vi "Motor_Lumicks_MengRonen.vi"() -> ()   [LabVIEW 2014]
uses:
  <vilib>/userdefined/High Color/IMAQdx.ctl
  <vilib>/Utility/inputDevices.llb/joystickAcquire.vi
  <vilib>/Utility/inputDevices.llb/closeJoystick.vi
  <vilib>/vision/driver/NI_Vision_Acquisition_Software.lvlib
panel:
  out "0 Position":T1={"X Pos (mm)"=2.683244, "Y Pos (mm)"=-0.037109375, "Z Pos (mm)"=0.2016383} {"Y Pos (mm)" format="%.3f"; "Z Pos (mm)" format="%.3f"; "X Pos (mm)" format="%.3f"}
  out "error out 2":errorcluster
  out "Image":T2(plugin-control)
  in  "Goto Channel 5":bool
  in  "Goto Channel 4":bool
  in  "Capture Channel 5":bool
  in  "Capture Channel 4":bool
  out "Channel 5":T1={"X Pos (mm)"=0.00014575559, "Y Pos (mm)"=-0.0013701026, "Z Pos (mm)"=0.004635028} {"Y Pos (mm)" format="%.3f"; "Z Pos (mm)" format="%.3f"; "X Pos (mm)" format="%.3f"}
  out "Channel 4":T1={"X Pos (mm)"=0.00014575559, "Y Pos (mm)"=-0.0013701026, "Z Pos (mm)"=0.004635028} {"Y Pos (mm)" format="%.3f"; "Z Pos (mm)" format="%.3f"; "X Pos (mm)" format="%.3f"}
  in  "Stop All":bool=TRUE
  out "button 4":bool
  in  "button 3":bool
  in  "Motor Cruise Param":T3={"X Acc (mm/s^2)"=0.1, "X Vmax (mm/s)"=1.0, "Y Acc (mm/s^2)"=0.3, "Y Vmax (mm/s)"=1.0, "Z Acc (mm/s^2)"=0.1, "Z Vmax (mm/s)"=0.1}
  out "XYZ position":sgl[](array[numeric])=[1.7793261, 1.7925023, 3.857043]
  in  "Motor Limits":T4={"XMAX"=12.0, "XMIN"=-12.0, "YMAX"=12.0, "YMIN"=-12.0, "ZMAX"=10.0, "ZMIN"=-10.0}
  in  "Motor settings (X,Y)":cluster{"Vmax (mm/s)":sgl, "Acc (mm/s/s)":sgl}={"Vmax (mm/s)"=0.05, "Acc (mm/s/s)"=0.2}
  in  "Motor settings (Z)":cluster{"Vmax (mm/s)":sgl, "Acc (mm/s/s)":sgl}={"Vmax (mm/s)"=0.02, "Acc (mm/s/s)"=0.2}
  in  "Capture Channel 3":bool
  in  "Capture Channel 2":bool
  in  "Capture Channel 1":bool
  in  "Goto Channel 2":bool
  in  "Goto Channel 3":bool
  in  "Goto Channel 1":bool
  out "Channel 1":T1={"X Pos (mm)"=2.683244, "Y Pos (mm)"=-0.037109375, "Z Pos (mm)"=0.2016383} {"Y Pos (mm)" format="%.3f"; "Z Pos (mm)" format="%.3f"; "X Pos (mm)" format="%.3f"}
  out "Channel 2":T1={"X Pos (mm)"=2.3714144, "Y Pos (mm)"=-0.4775245, "Z Pos (mm)"=0.20615672} {"Y Pos (mm)" format="%.3f"; "Z Pos (mm)" format="%.3f"; "X Pos (mm)" format="%.3f"}
  out "Channel 3":T1={"X Pos (mm)"=3.6928055, "Y Pos (mm)"=-0.788188, "Z Pos (mm)"=0.19962686} {"Y Pos (mm)" format="%.3f"; "Z Pos (mm)" format="%.3f"; "X Pos (mm)" format="%.3f"}
  out "error out":errorcluster
  in  "MG17Motor Z":refnum<k7>(container)
  in  "MG17Motor Y":refnum<k7>(container)
  in  "MG17Motor X":refnum<k7>(container)
  out "Stage Moving":bool
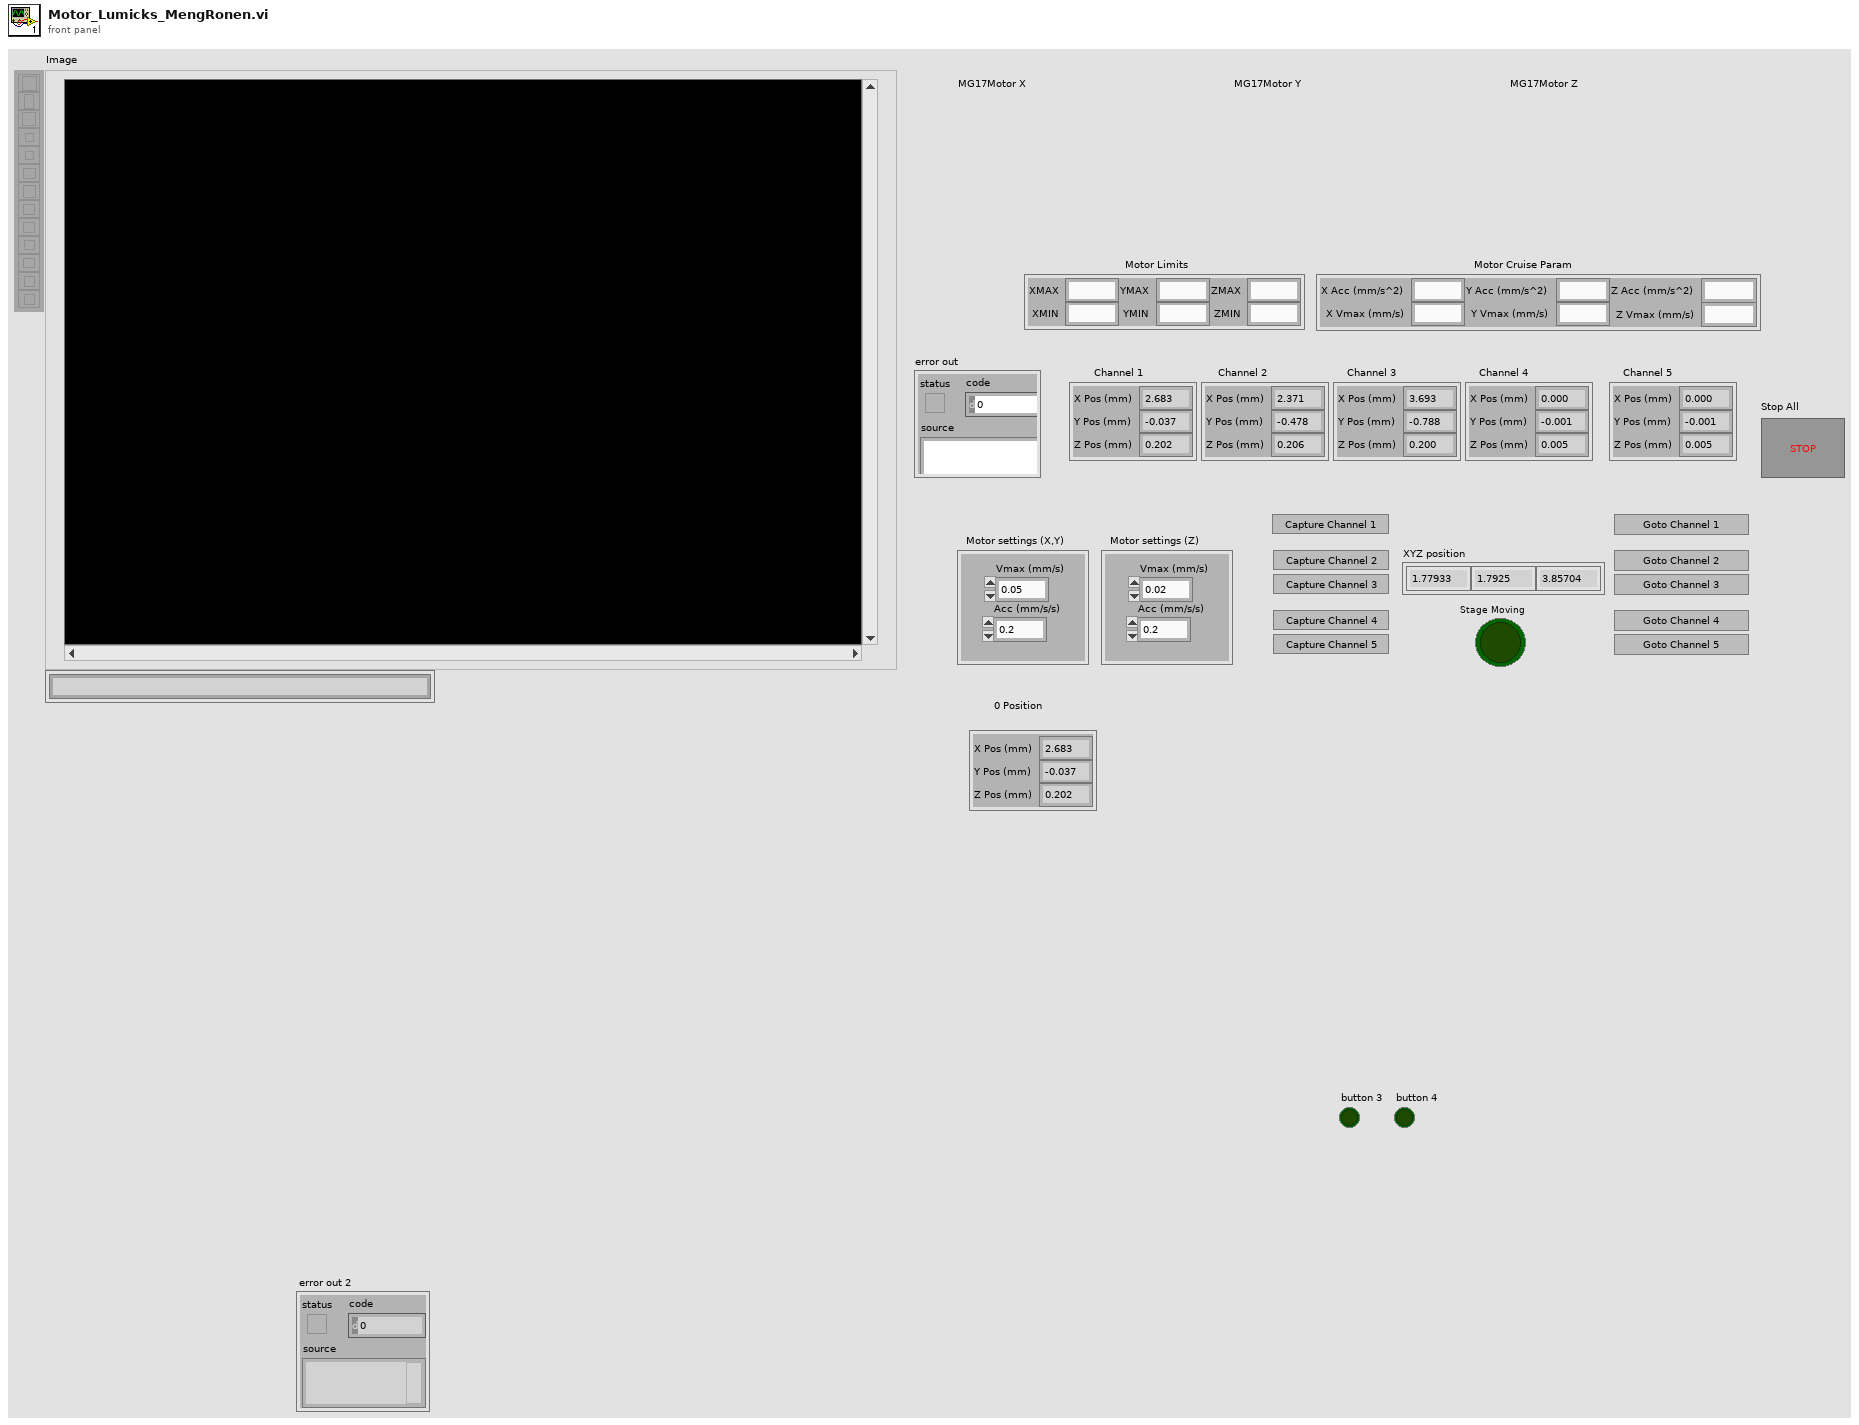
[diagram p1: front panel]
types:
  T1 = cluster{"X Pos (mm)":sgl, "Y Pos (mm)":sgl, "Z Pos (mm)":sgl}
  T2 = typedef "IMAQ Image.ctl" = refnum<image>
  T3 = cluster{"X Acc (mm/s^2)":sgl, "X Vmax (mm/s)":sgl, "Y Acc (mm/s^2)":sgl, "Y Vmax (mm/s)":sgl, "Z Acc (mm/s^2)":sgl, "Z Vmax (mm/s)":sgl}
  T4 = cluster{"XMAX":sgl, "XMIN":sgl, "YMAX":sgl, "YMIN":sgl, "ZMAX":sgl, "ZMIN":sgl}
  T5 = typedef "IMAQdx.ctl" = refnum<k21>
  T6 = typedef "Image Type" = u32
  T7 = cluster{"X axis":i32, "Y axis":i32, "Z axis":i32, "X axis rotation":i32, "Y axis rotation":i32, "Z axis rotation":i32, "U axis":i32, "V axis":i32}
  T8 = cluster{"button 1":bool, "button 2":bool, "button 3":bool, "button 4":bool, "button 5":bool, "button 6":bool, "button 7":bool, "button 8":bool, "button 9":bool, "button 10":bool, "button 11":bool, "button 12":bool, "button 13":bool, "button 14":bool, "button 15":bool, "button 16":bool, "button 17":bool, "button 18":bool, "button 19":bool, "button 20":bool, "button 21":bool, "button 22":bool, "button 23":bool, "button 24":bool, "button 25":bool, "button 26":bool, "button 27":bool, "button 28":bool, "button 29":bool, "button 30":bool, "button 31":bool, "button 32":bool}
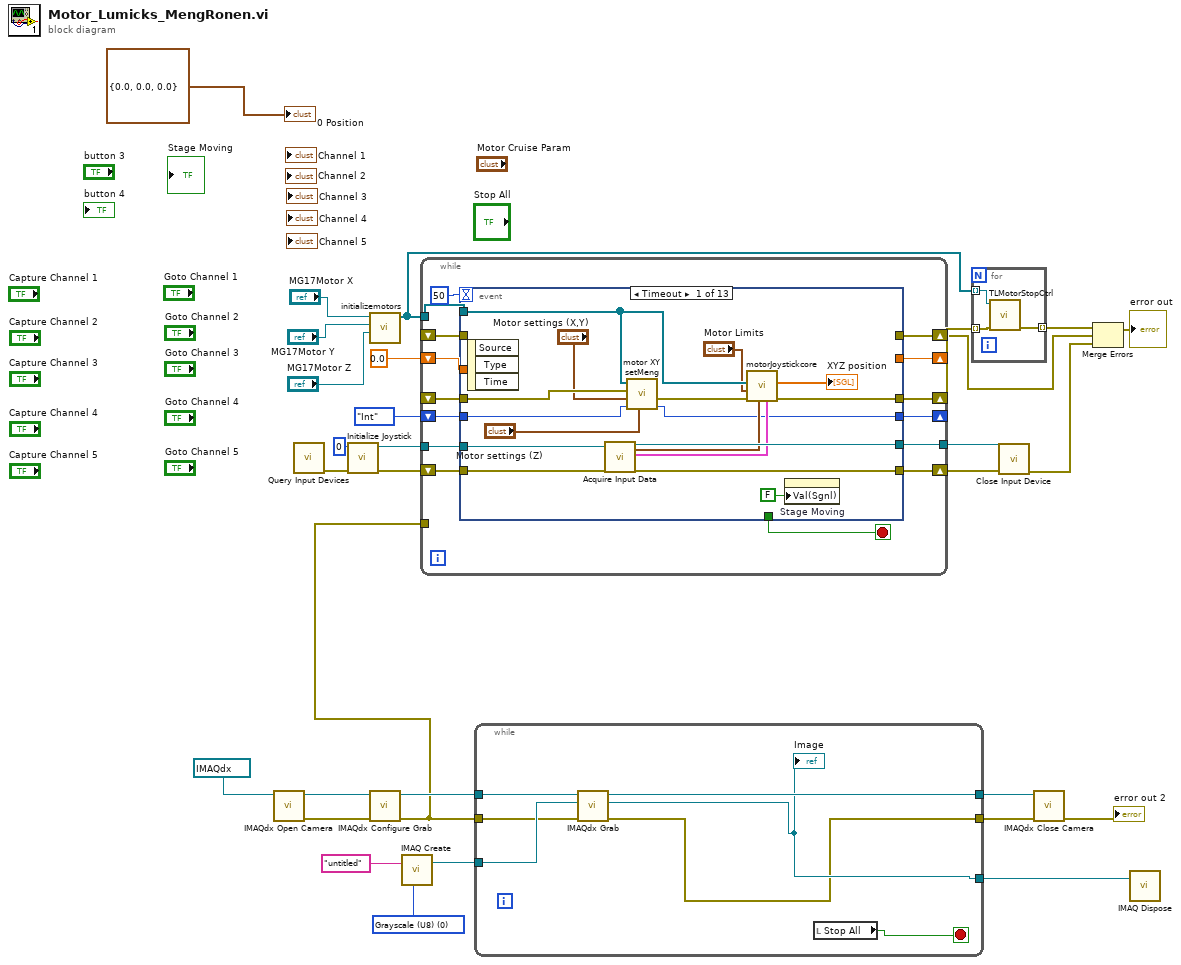
[diagram p0: block diagram]
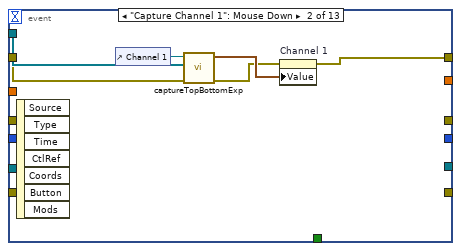
[diagram p2: hidden frame]
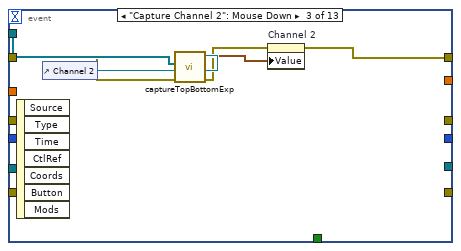
[diagram p3: hidden frame]
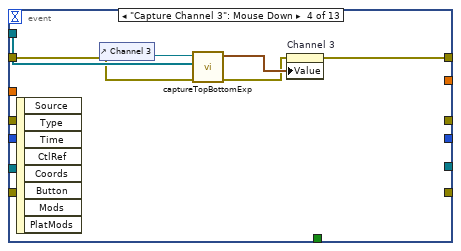
[diagram p4: hidden frame]
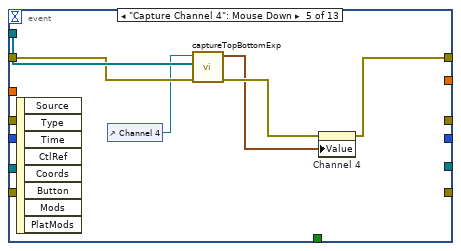
[diagram p5: hidden frame]
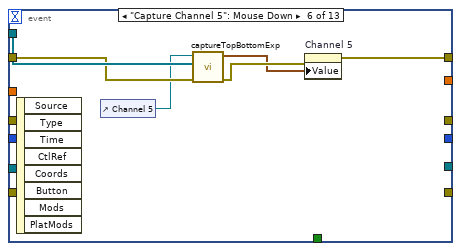
[diagram p6: hidden frame]
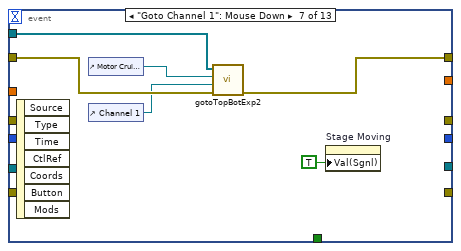
[diagram p7: hidden frame]
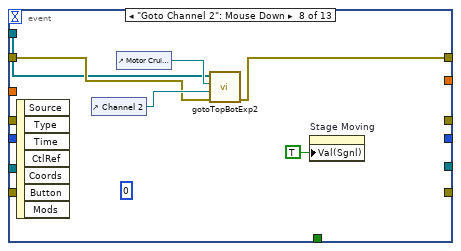
[diagram p8: hidden frame]
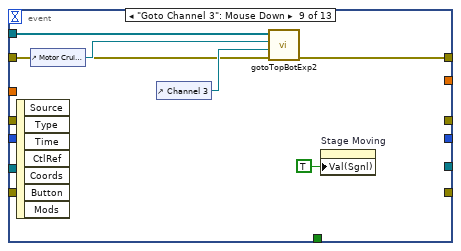
[diagram p9: hidden frame]
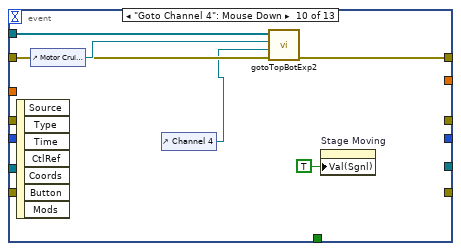
[diagram p10: hidden frame]
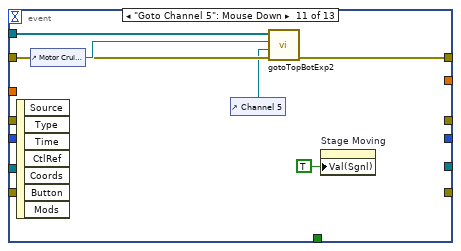
[diagram p11: hidden frame]
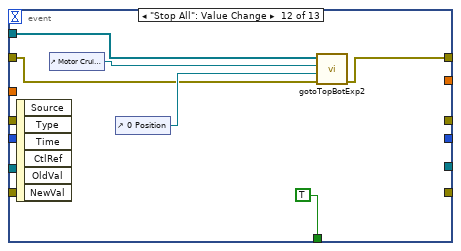
[diagram p12: hidden frame]
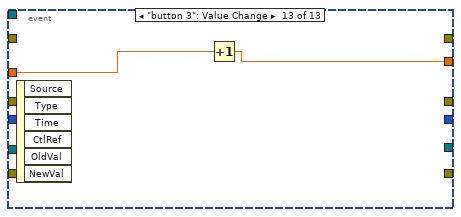
[diagram p13: hidden frame]
diagram:
  w7 = T6 0 items=["Grayscale (U8)", "Grayscale (I16)", "Grayscale (SGL)", "Complex (CSG)", "RGB (U32)", "HSL (U32)", "RGB (U64)", "Grayscale (U16)"] ("Image Type")
  n1 = call <vilib>:"IMAQdx Open Camera.vi"("Session In"=T5 "cam0") -> ("error out"=w11:errorcluster, "Session Out"=w10:T5)  [unwired: 9 in]
  n2 = call <vilib>:"Query Input Devices.vi"() -> ("error out"=w23:errorcluster)  [unwired: 8 in, 3 out]
  n3 = call <vilib>:"Initialize Joystick.vi"("error in (no error)"=w23, "device index"=0) -> ("error out"=w20:errorcluster, "device ID"=w21:refnum<k1>)  [unwired: 8 in]
  n4 = call "initializemotors.vi"("MG17Motor Z"="MG17Motor Z", "MG17Motor Y"="MG17Motor Y", "Automation Refnum in"="MG17Motor X") -> ("Array 2"=w25:refnum<k7>[])  [unwired: 7 in, 1 out]
  n5 = call <vilib>:"IMAQdx Configure Grab.vi"("error in"=w11, "Session In"=w10) -> ("error out"=w2:errorcluster, "Session Out"=w9:T5)  [unwired: 8 in]
  n6 = call "IMAQ Create"("Image Name"="untitled", "Image Type"=w7) -> ("New Image"=w13:T2)  [unwired: 3 in, 1 out]
  n7 = while {
    tunnel: w25 -> [w45]
    shift-right: [w44] -> w15
    shift-left: _ -> [w43]
    shift-right: [w40] -> _
    shift-left: 0.0 -> [w41]
    tunnel: w21 -> [w39]
    shift-right: [w37] -> w19
    shift-left: w20 -> [w38]
    tunnel: [w36] -> w18
    shift-right: [w35] -> w16
    shift-left: _ -> [w34]
    shift-right: [w32] -> _
    shift-left: enum16{"Int", "Set"}."Int" ("Enum") -> [w33]
    tunnel: w2 -> [_]
    stop <- w42 stop-if-true
    n8 = event shown="[0] Timeout" {
      selector: _ -> [_ _ _ _ _ _ _ _ _ _ _ _ _]
      dyn-events: _ -> [_ _ _ _ _ _ _ _ _ _ _ _ _]
      timeout: 50 -> [_ _ _ _ _ _ _ _ _ _ _ _ _]
      tunnel: w45 -> [w52 w68 w73 w80 w86 w92 w94 w100 w106 w113 w119 w124 _]
      tunnel: [_ w65 w69 w75 w82 w87 w97 w101 w107 w114 w120 w125 _] -> w44
      tunnel: w43 -> [_ w64 w72 w78 w85 w91 w98 w102 w108 w115 w121 w126 _]
      tunnel: [_ _ _ _ _ _ _ _ _ _ _ TRUE _] -> w42
      tunnel: [_ _ _ _ _ _ _ _ _ _ _ _ w130] -> w40
      tunnel: w41 -> [_ _ _ _ _ _ _ _ _ _ _ _ w129]
      tunnel: w39 -> [w62 _ _ _ _ _ _ _ _ _ _ _ _]
      tunnel: w38 -> [w61 _ _ _ _ _ _ _ _ _ _ _ _]
      tunnel: [w60 _ _ _ _ _ _ _ _ _ _ _ _] -> w37
      tunnel: [w59 _ _ _ _ _ _ _ _ _ _ _ _] -> w36
      tunnel: [w55 _ _ _ _ _ _ _ _ _ _ _ _] -> w35
      tunnel: w34 -> [w54 _ _ _ _ _ _ _ _ _ _ _ _]
      tunnel: w33 -> [w48 _ _ _ _ _ _ _ _ _ _ _ _]
      tunnel: [w47 _ _ _ _ _ _ _ _ _ _ _ _] -> w32
      event Timeout {
        n9 = event-data() -> ()  [unwired: 1 in, 3 out]
        n10 = call-poly <vilib>:"Acquire Input Data.vi"("device ID"=w62, "error in (no error)"=w61) -> ("device ID"=w59:refnum<k1>, "axis info"=w57:T7, "button info"=w58:T8, "error out"=w60:errorcluster)  [unwired: 13 in, 1 out]
        n11 = call "motor XY setMeng.vi"("Motor settings Z"="Motor settings (Z)", "Enum in"=w48, "Motor settings (X,Y)"="Motor settings (X,Y)", "Array"=w54, "Array 2"=w52) -> ("Enum out"=w47:enum16{"Int", "Set"}, "Array 3"=w53:errorcluster[])  [unwired: 4 in, 1 out]
        n12 = call "motorJoystickcore.vi"("button info"=w58, "axis info"=w57, "error in"=w53, "Motor Limits"="Motor Limits", "Array in"=w52) -> ("error out"=w55:errorcluster[], "XYZ position"=→"XYZ position":sgl[])  [unwired: 5 in]
        n13 = property on="Stage Moving" class="Bool (strict)"("Val(Sgnl)"=FALSE ("Value (Signaling)")) -> ()  [unwired: 2 in, 2 out]
      }
      event "Capture Channel 1": Mouse Down {
        n14 = event-data() -> ()  [unwired: 1 in, 7 out]
        n15 = control-ref of="Channel 1"() -> (w63:refnum<vi>)
        n16 = call "captureTopBottomExp.vi"("error in (no error)"=w64, "Array in"=w68, "Cluster in"=w63) -> ("error out"=w66:errorcluster, "Value"=w67:T1)  [unwired: 7 in]
        n17 = property on="Channel 1" class="Clust (strict)"(error in=w66, "Value"=w67) -> (error out=w65:errorcluster)  [unwired: 1 in, 1 out]
      }
      event "Capture Channel 2": Mouse Down {
        n18 = event-data() -> ()  [unwired: 1 in, 7 out]
        n19 = control-ref of="Channel 2"() -> (w74:refnum<vi>)
        n20 = call "captureTopBottomExp.vi"("error in (no error)"=w72, "Array in"=w73, "Cluster in"=w74) -> ("error out"=w70:errorcluster, "Value"=w71:T1)  [unwired: 7 in]
        n21 = property on="Channel 2" class="Clust (strict)"(error in=w70, "Value"=w71) -> (error out=w69:errorcluster)  [unwired: 1 in, 1 out]
      }
      event "Capture Channel 3": Mouse Down {
        n22 = event-data() -> ()  [unwired: 1 in, 8 out]
        n23 = control-ref of="Channel 3"() -> (w79:refnum<vi>)
        n24 = call "captureTopBottomExp.vi"("error in (no error)"=w78, "Array in"=w80, "Cluster in"=w79) -> ("error out"=w76:errorcluster, "Value"=w77:T1)  [unwired: 7 in]
        n25 = property on="Channel 3" class="Clust (strict)"(error in=w76, "Value"=w77) -> (error out=w75:errorcluster)  [unwired: 1 in, 1 out]
      }
      event "Capture Channel 4": Mouse Down {
        n26 = event-data() -> ()  [unwired: 1 in, 8 out]
        n27 = control-ref of="Channel 4"() -> (w84:refnum<vi>)
        n28 = call "captureTopBottomExp.vi"("error in (no error)"=w85, "Array in"=w86, "Cluster in"=w84) -> ("error out"=w83:errorcluster, "Value"=w81:T1)  [unwired: 7 in]
        n29 = property on="Channel 4" class="Clust (strict)"(error in=w83, "Value"=w81) -> (error out=w82:errorcluster)  [unwired: 1 in, 1 out]
      }
      event "Capture Channel 5": Mouse Down {
        n30 = event-data() -> ()  [unwired: 1 in, 8 out]
        n31 = control-ref of="Channel 5"() -> (w90:refnum<vi>)
        n32 = call "captureTopBottomExp.vi"("error in (no error)"=w91, "Array in"=w92, "Cluster in"=w90) -> ("error out"=w89:errorcluster, "Value"=w88:T1)  [unwired: 7 in]
        n33 = property on="Channel 5" class="Clust (strict)"(error in=w89, "Value"=w88) -> (error out=w87:errorcluster)  [unwired: 1 in, 1 out]
      }
      event "Goto Channel 1": Mouse Down {
        n34 = event-data() -> ()  [unwired: 1 in, 7 out]
        n35 = control-ref of="Motor Cruise Param"() -> (w96:refnum<vi>)
        n36 = control-ref of="Channel 1"() -> (w95:refnum<vi>)
        n37 = call "gotoTopBotExp2.vi"("error in (no error)"=w98, "position"=w95, "motor setting"=w96, "appended array"=w94) -> ("error out"=w97:errorcluster)  [unwired: 7 in]
        n38 = property on="Stage Moving" class="Bool (strict)"("Val(Sgnl)"=TRUE ("Value (Signaling)")) -> ()  [unwired: 2 in, 2 out]
      }
      event "Goto Channel 2": Mouse Down {
        (unwired) 0 ("lChanID")
        n39 = event-data() -> ()  [unwired: 1 in, 7 out]
        n40 = control-ref of="Channel 2"() -> (w103:refnum<vi>)
        n41 = control-ref of="Motor Cruise Param"() -> (w104:refnum<vi>)
        n42 = call "gotoTopBotExp2.vi"("error in (no error)"=w102, "position"=w103, "motor setting"=w104, "appended array"=w100) -> ("error out"=w101:errorcluster)  [unwired: 7 in]
        n43 = property on="Stage Moving" class="Bool (strict)"("Val(Sgnl)"=TRUE ("Value (Signaling)")) -> ()  [unwired: 2 in, 2 out]
      }
      event "Goto Channel 3": Mouse Down {
        n44 = event-data() -> ()  [unwired: 1 in, 7 out]
        n45 = control-ref of="Motor Cruise Param"() -> (w110:refnum<vi>)
        n46 = control-ref of="Channel 3"() -> (w109:refnum<vi>)
        n47 = call "gotoTopBotExp2.vi"("error in (no error)"=w108, "position"=w109, "motor setting"=w110, "appended array"=w106) -> ("error out"=w107:errorcluster)  [unwired: 7 in]
        n48 = property on="Stage Moving" class="Bool (strict)"("Val(Sgnl)"=TRUE ("Value (Signaling)")) -> ()  [unwired: 2 in, 2 out]
      }
      event "Goto Channel 4": Mouse Down {
        n49 = event-data() -> ()  [unwired: 1 in, 7 out]
        n50 = control-ref of="Motor Cruise Param"() -> (w116:refnum<vi>)
        n51 = control-ref of="Channel 4"() -> (w111:refnum<vi>)
        n52 = call "gotoTopBotExp2.vi"("error in (no error)"=w115, "position"=w111, "motor setting"=w116, "appended array"=w113) -> ("error out"=w114:errorcluster)  [unwired: 7 in]
        n53 = property on="Stage Moving" class="Bool (strict)"("Val(Sgnl)"=TRUE ("Value (Signaling)")) -> ()  [unwired: 2 in, 2 out]
      }
      event "Goto Channel 5": Mouse Down {
        n54 = event-data() -> ()  [unwired: 1 in, 7 out]
        n55 = control-ref of="Motor Cruise Param"() -> (w122:refnum<vi>)
        n56 = control-ref of="Channel 5"() -> (w117:refnum<vi>)
        n57 = call "gotoTopBotExp2.vi"("error in (no error)"=w121, "position"=w117, "motor setting"=w122, "appended array"=w119) -> ("error out"=w120:errorcluster)  [unwired: 7 in]
        n58 = property on="Stage Moving" class="Bool (strict)"("Val(Sgnl)"=TRUE ("Value (Signaling)")) -> ()  [unwired: 2 in, 2 out]
      }
      event "Stop All": Value Change {
        n59 = event-data() -> ()  [unwired: 1 in, 6 out]
        n60 = control-ref of="Motor Cruise Param"() -> (w123:refnum<vi>)
        n61 = control-ref of="0 Position"() -> (w127:refnum<vi>)
        n62 = call "gotoTopBotExp2.vi"("error in (no error)"=w126, "position"=w127, "motor setting"=w123, "appended array"=w124) -> ("error out"=w125:errorcluster)  [unwired: 7 in]
      }
      event "button 3": Value Change {
        n63 = event-data() -> ()  [unwired: 1 in, 6 out]
        n64 = Increment(x=w129) -> (x+1=w130:dbl)
      }
    }
  }
  n65 = while {
    tunnel: w13 -> [w136]
    tunnel: w9 -> [w137]
    tunnel: w2 -> [w135]
    tunnel: [w131] -> w6
    tunnel: [w134] -> w5
    tunnel: [w132] -> w3
    stop <- w133 stop-if-true
    n66 = call <vilib>:"IMAQdx Grab.vi"("error in"=w135, "Image In"=w136, "Session In"=w137) -> ("error out"=w131:errorcluster, "Image Out"=w132:T2, "Session Out"=w134:T5)  [unwired: 5 in, 1 out]
    "Image" <- w132
    n67 = local read "Stop All"() -> (w133:bool)
  }
  n68 = for {
    tunnel: w25 -> [w140] mode=indexing
    tunnel: w16 -> [w139] mode=indexing
    tunnel: [w138] -> w27 mode=indexing
    n69 = call "TLMotorStopCtrl.vi"("Error In (No Error)"=w139, "Motor Ref"=w140) -> ("Error Out"=w138:errorcluster)  [unwired: 4 in, 1 out]
  }
  n70 = call-poly <vilib>:"Close Input Device.vi"("error in (no error)"=w19, "device ID"=w18) -> ("error out"=w14:errorcluster)  [unwired: 8 in]
  n71 = call <vilib>:"IMAQdx Close Camera.vi"("error in"=w6, "Session In"=w5) -> ("error out"=→"error out 2":errorcluster)  [unwired: 9 in]
  n72 = Merge Errors(w27, w15, w14) -> (→"error out":errorcluster)
  n73 = call "IMAQ Dispose"("Image"=w3) -> ()  [unwired: 5 in, 1 out]
  "0 Position" <- cluster{dbl, dbl, dbl} {0.0, 0.0, 0.0}
